vi "Set Index.vi"(8 "Error In":errorcluster, 10 "Index":u16, 11 "reference in":refnum<class "OD Entry.lvclass">) -> (0 "Error Out":errorcluster, 3 "reference out":refnum<class "OD Entry.lvclass">)   [LabVIEW 2024, in "Electronic Datasheet.lvlib" / "OD Entry.lvclass"]
uses:
  OD Entry.lvclass
  OD Entry.lvclass/OD Entry.ctl
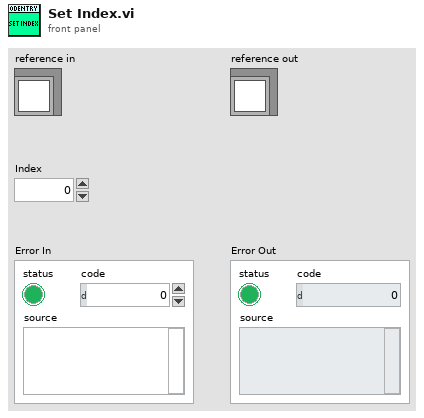
[diagram p1: front panel]
types:
  T1 = typedef "Electronic Datasheet.lvlib/OD Entry.lvclass/ObjectAttributes.ctl" = cluster{"Index":u16, "ObjectType":refnum<class "Object Type Base.lvclass">, "Denotation":string, "Count":u8, "ObjExtend":u8, "PDOtype":T2, "Label":string, "Description":string, "Sub-Entries":map{u8, refnum<class "OD Sub-Entry.lvclass">}}
  T2 = typedef "Electronic Datasheet.lvlib/PDO Mapping Type.ctl" = enum16{"NO", "OPTIONAL", "RPDO", "TPDO", "DEFAULT"}
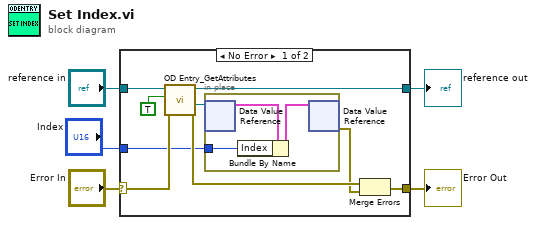
[diagram p0: block diagram]
diagram:
  n1 = case shown="No Error" "Error In" {
    selector: "Error In" -> [w13 w19]
    tunnel: [w14 w19] -> w4
    tunnel: [w10 w18] -> w2
    tunnel: "reference in" -> [w11 w18]
    tunnel: "Index" -> [w7 _]
    frame No Error {
      n2 = call "OD Entry_GetAttributes.vi"("Error In"=w13, "OnlyGetDvrReference(False)"=TRUE, "reference in"=w11) -> ("Error Out"=w12:errorcluster, "DataRef"=w8:refnum<data-value>, "reference out"=w10:refnum<class "OD Entry.lvclass">)  [unwired: 5 in, 1 out]
      n3 = in-place {
        in-place-border: w7 -> [w17]
        n4 = in-place-dvr #1(w8) -> (w16:T1)  [unwired: 1 out]
        n5 = Bundle By Name(cluster=w16, "Index"=w17) -> (w15:T1)
        n6 = in-place-dvr #1(w15) -> (w6:errorcluster)  [unwired: 1 out]
      }
      n7 = Merge Errors(w12, w6) -> (w14:errorcluster)
    }
    frame Error {
    }
  }
  "Error Out" <- w4
  "reference out" <- w2
